vi "From.vi"(1 "Value":bool=TRUE) -> (0 "Boolean":refnum<class "Boolean.lvclass">)   [LabVIEW 2018, in "Toolkit.lvlib" / "Types.lvlib" / "Boolean.lvclass"]
doc: "Wraps a LabVIEW boolean primitative value in a Mustache data type object."
uses:
  Boolean.lvclass
  Boolean.lvclass/Boolean.ctl
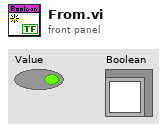
[diagram p1: front panel]
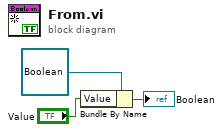
[diagram p0: block diagram]
diagram:
  n1 = Bundle By Name(cluster=refnum<class "Boolean.lvclass"> refnum ("Toolkit.lvlib:Data.lvlib:Boolean.lvclass"), "Value"="Value") -> (→"Boolean":refnum<class "Boolean.lvclass">)
